vi "Start Cooking Recipe.vi"(8 "error in (no error)":errorcluster, 10 "Recipe":string[][](table), 11 "Kitchen Actor in":refnum<class "Kitchen Actor.lvclass">) -> (0 "error out":errorcluster, 3 "Kitchen Actor out":refnum<class "Kitchen Actor.lvclass">)   [LabVIEW 2021, in "Kitchen Actor.lvlib" / "Kitchen Actor.lvclass"]
uses:
  Kitchen Actor.lvclass
  Cooker Actor/Cooker Actor Messages/Start Cooking Recipe Msg/Start Cooking Recipe Msg.lvclass
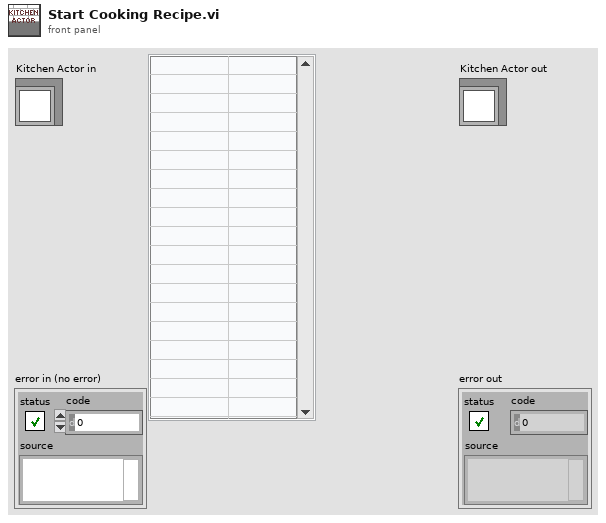
[diagram p1: front panel]
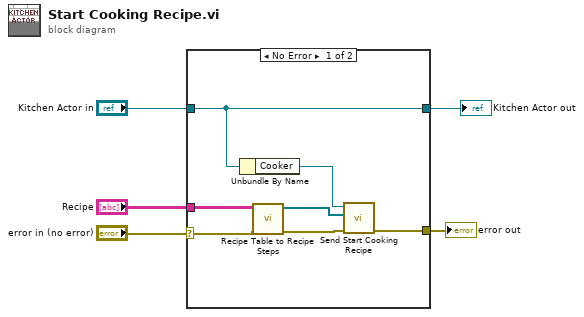
[diagram p0: block diagram]
diagram:
  n1 = case shown="No Error" "error in (no error)" {
    selector: "error in (no error)" -> [w7 w14]
    tunnel: [w10 w14] -> w4
    tunnel: [w12 w13] -> w2
    tunnel: "Kitchen Actor in" -> [w12 w13]
    tunnel: "Recipe" -> [w8 _]
    frame No Error {
      n2 = Unbundle By Name(w12) -> ("Cooker"=w11:refnum<class "Message Enqueuer.lvclass">)
      n3 = call "Recipe Table to Recipe Steps.vi"("error in (no error)"=w7, "Recipe"=w8) -> ("error out"=w6:errorcluster, "Recipe Steps"=w9:refnum<class "Recipe Step.lvclass">[])  [unwired: 8 in]
      n4 = call "Send Start Cooking Recipe.vi"("error in (no error)"=w6, "Steps"=w9, "Message Enqueuer"=w11) -> ("error out"=w10:errorcluster)  [unwired: 7 in, 1 out]
    }
    frame Error {
    }
  }
  "error out" <- w4
  "Kitchen Actor out" <- w2
